vi "LEIN CMD create ACTI.vi"(0 "SID":u8, 1 "LEIN Variation":T1=enum."LEIN63", 5 "Data":u8[](array[numeric]), 7 "ACTI ID":u8, 11 "error in (no error)":errorcluster) -> (8 "CMD":T2={"SID"=0, "ANF"=FALSE, "CMD"=enum."TASK", "DATA"=[]}, 15 "error out":errorcluster)   [LabVIEW 2011]
uses:
  Defenitions/LEIN CMD Cluster.ctl
  Defenitions/LEIN CMD List.ctl
  Defenitions/LEIN Structure variations.ctl
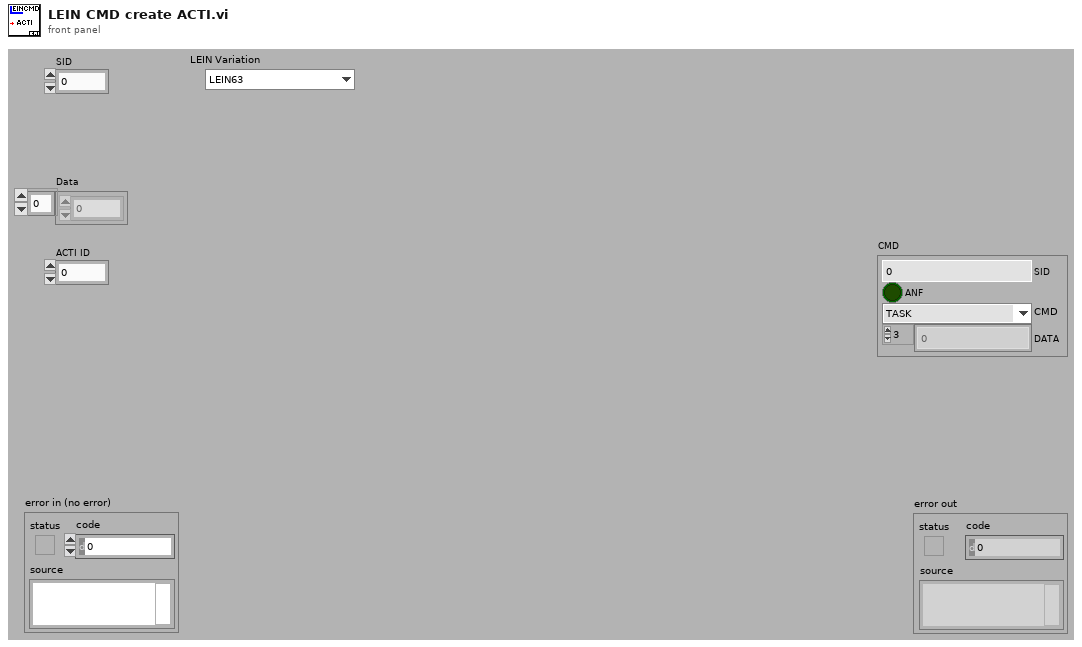
[diagram p1: front panel]
types:
  T1 = typedef "LEIN Structure variations.ctl" = enum16{"LEIN08", "LEIN31", "LEIN63"}
  T2 = typedef "LEIN CMD Cluster.ctl" = cluster{"SID":u8, "ANF":bool, "CMD":T3, "DATA":u8[]}
  T3 = typedef "LEIN CMD List.ctl" = enum8{"ACTI", "TASK", "RES0", "STAT", "RES1", "RES2", "RES3", "USER"}
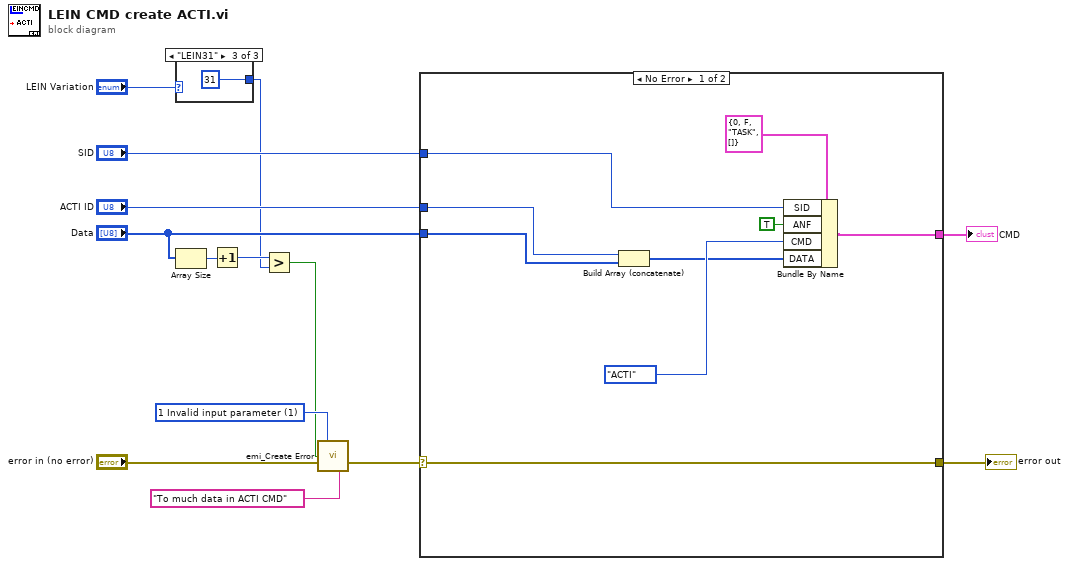
[diagram p0: block diagram]
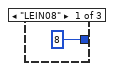
[diagram p2: hidden frame]
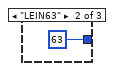
[diagram p3: hidden frame]
diagram:
  w14 = 1 items=["0 No Error"=0, "1 Invalid input parameter"=1, "6 Generic file IO "=6, "7 File not Found"=7, "35 Generic Pring Error"=35, "37 Device not Found"=37, "39 Device Unit Error"=39, "40 Could fot Open Device"=40, "42 Generic Error"=42, "52 Unknown Message"=52, "98 Bad File type"=98, "99 Bad File Version"=99, "100 Bad Data in File"=100, "1018 Unspecefied Error"=1018, "1041 Incorrect Password"=1041, "1043 Feature not in this version"=1043, "1109 Unsuported Data type"=1109, "1444 Did not close sucessfully"=1444] ("Error Code")
  n1 = case shown="\"LEIN31\"" "LEIN Variation" {
    tunnel: [8 ("y") 63 ("y") 31 ("y")] -> w2
    frame "LEIN08" {
    }
    frame "LEIN63" {
    }
    frame "LEIN31" {
    }
  }
  n2 = Array Size(array="Data") -> (size(s)=w4:i32)
  n3 = Increment(x=w4) -> (x+1=w3:i32)
  n4 = Greater?(x=w3, y=w2) -> (0:w1:bool)
  n5 = call "emi_Create Error.vi"("Error Code"=w14, "Error(T)"=w1, "error in (no error)"="error in (no error)", "Append String(\"\")"="To much data in ACTI CMD" ("Append String(\"\")")) -> ("error out"=w12:errorcluster)  [unwired: 11 in]
  n6 = case shown="No Error" w12 {
    selector: w12 -> [w26 w27]
    tunnel: [w26 w27] -> w10
    tunnel: "ACTI ID" -> [w18 _]
    tunnel: "Data" -> [w19 _]
    tunnel: [w24 _] -> w8
    tunnel: "SID" -> [w23 _]
    frame No Error {
      n7 = Build Array (concatenate)(w18, w19) -> (w20:u8[])
      n8 = Bundle By Name(cluster=T2 {"SID"=0, "ANF"=FALSE, "CMD"=enum."TASK", "DATA"=[]} ("CMD"), "SID"=w23, "ANF"=TRUE, "CMD"=LEIN_CMD_List."ACTI", "DATA"=w20) -> (w24:T2)
    }
    frame Error {
    }
  }
  "error out" <- w10
  "CMD" <- w8
